vi "CRYTS Step Unflatten Lib.vi"(9 "Version":i32, 10 "Sequence Name":string, 11 "Steps In":T1[](array[typedef]) {"Repeat State Array"."Start" format="%#_5g"; "Y dB ref" format="%.1f"; "Y data" items=["dB", "Lin"]; "Start" format="%#_5g"}) -> (3 "Steps Out":T1[](array[typedef]) {"Repeat State Array"."Start" format="%#_5g"; "Y dB ref" format="%.1f"; "Y data" items=["dB", "Lin"]; "Start" format="%#_5g"})   [LabVIEW 2013]
uses:
  CRYSystem/Typedef Control/CRYStep.ctl
  CRYSystem/Typedef Control/CRYStart Cluster.ctl
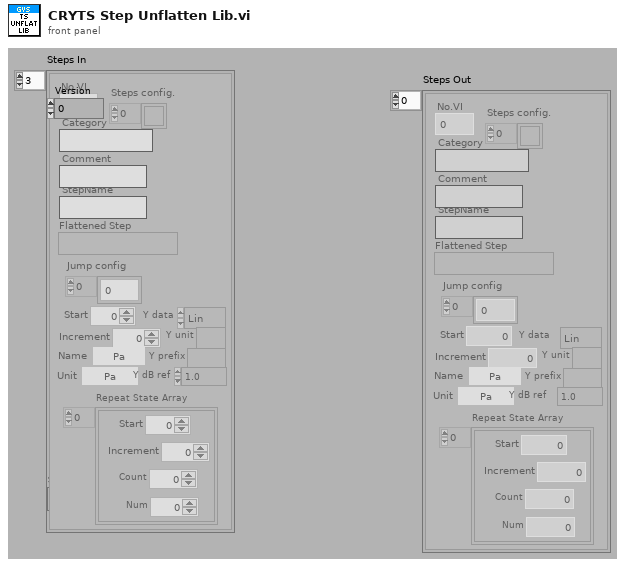
[diagram p1: front panel]
types:
  T1 = typedef "CRYStep.ctl" = cluster{"No.VI":i32, "Category":string, "StepName":string, "Seq setup flattened":string, "Comment":string, "Steps config.":bool[], "Jump config":i32[], "Start":dbl, "Increment":dbl, "Name":string, "Unit":string, "Y data":u16, "Y prefix":string, "Y dB ref":dbl, "Y unit":string, "Repeat State Array":cluster{"Start":dbl, "Increment":dbl, "Count":i32, "Num":i32}[]}
  T2 = typedef "CRYStart Cluster.ctl" = cluster{"SequenceName":string, "Preload Stimulus":bool, "CloseOpenedDisplay":bool, "ClearMeasuredData":bool, "UpdateDisplayDuringRun":bool, "DisplayForConfirmation":bool, "HaltOnFail":bool, "UseSameHardware":bool, "UseSameCalibration":bool}
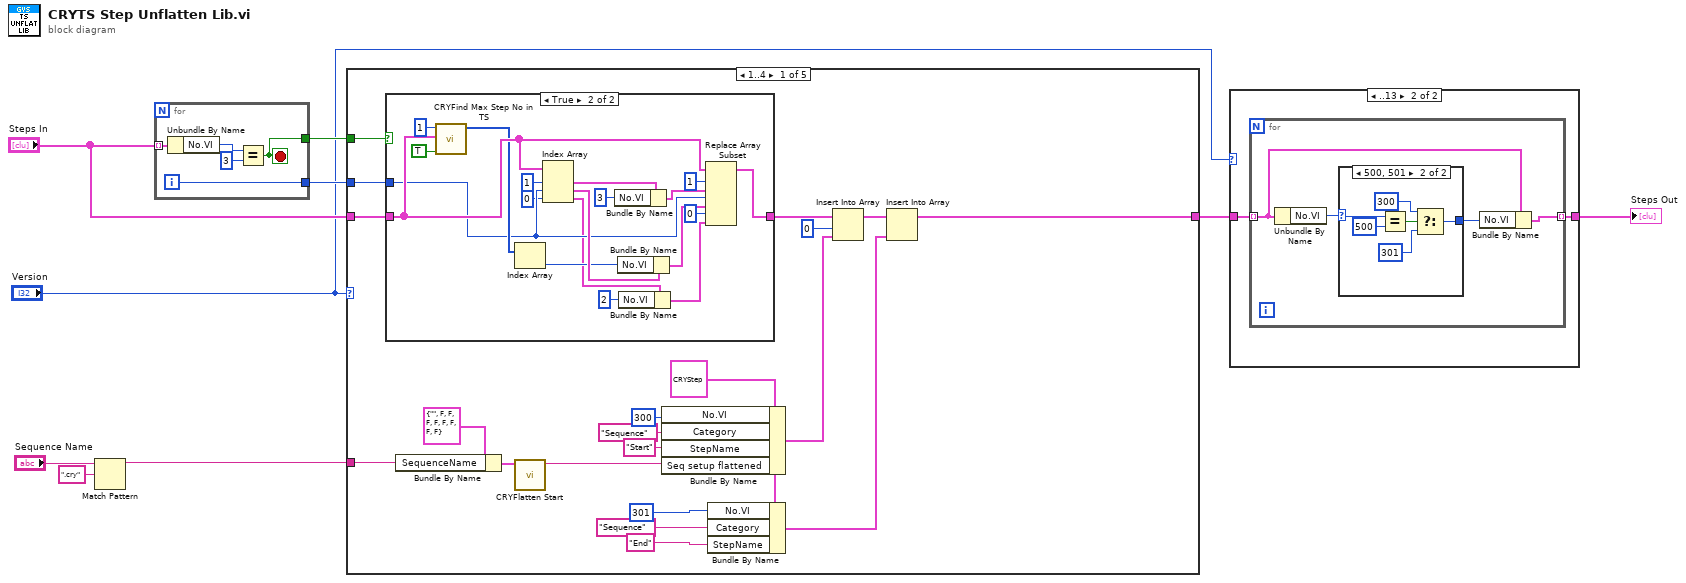
[diagram p0: block diagram]
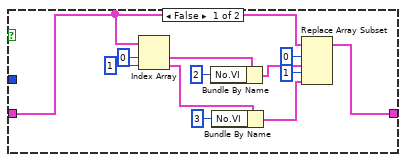
[diagram p4: hidden frame]
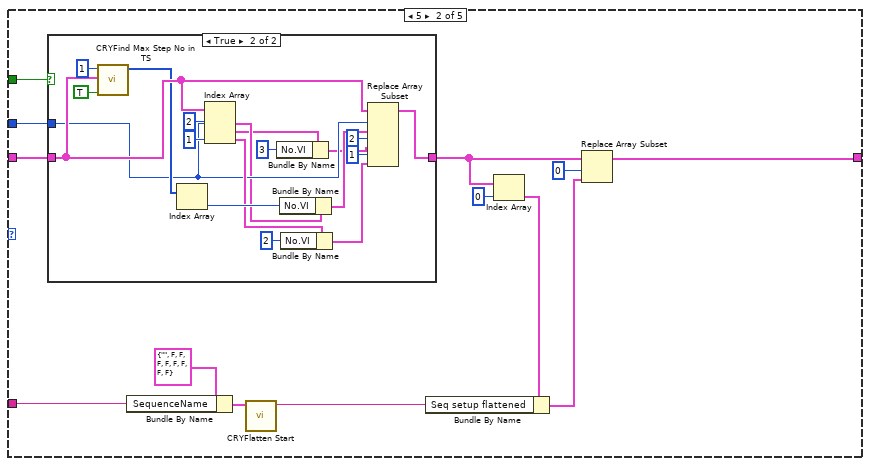
[diagram p5: hidden frame]
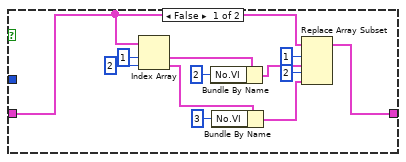
[diagram p6: hidden frame]
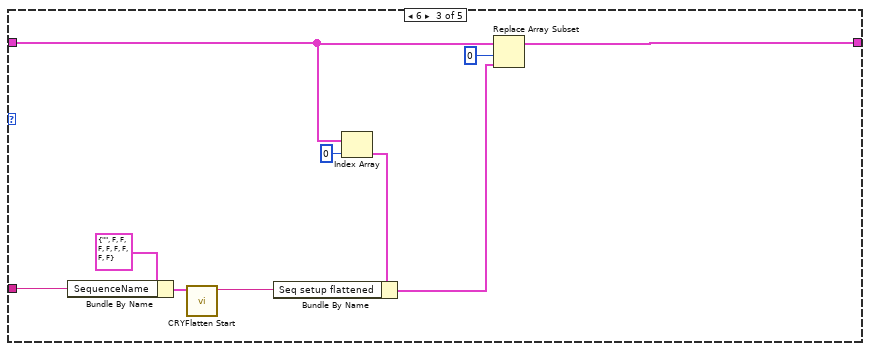
[diagram p7: hidden frame]
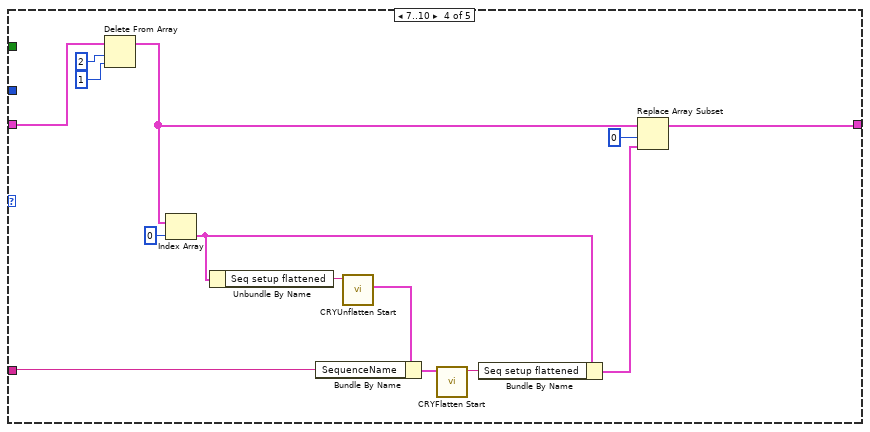
[diagram p8: hidden frame]
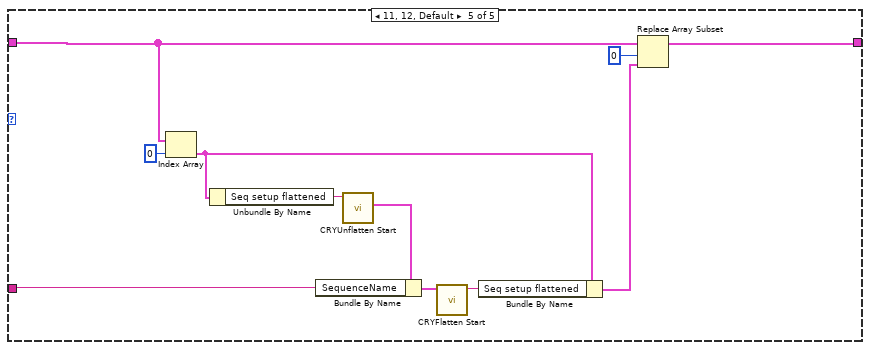
[diagram p9: hidden frame]
diagram:
  n1 = Match Pattern(string="Sequence Name", regular expression=".cry") -> (before substring=w4:string)  [unwired: 1 in, 3 out]
  n2 = for {
    tunnel: "Steps In" -> [w14] mode=indexing
    tunnel: [w11] -> w7
    tunnel: [w10] -> w9
    i -> [w11]
    stop <- w10 stop-if-true
    n3 = Unbundle By Name(w14) -> ("No.VI"=w13:i32)
    n4 = Equal?(x=w13, y=3) -> (x = y?=w10:bool)
  }
  n5 = case shown="1..4" "Version" {
    tunnel: w9 -> [w34 w76 _ _ _]
    tunnel: "Steps In" -> [w33 w78 w115 w123 w134]
    tunnel: w7 -> [w32 w77 _ _ _]
    tunnel: [w19 w70 w114 w130 w141] -> w2
    tunnel: w4 -> [w15 w67 w110 w126 w137]
    frame 1..4 {
      w29 = T1 {"No.VI"=0, "Category"="", "StepName"="", "Seq setup flattened"="", "Comment"="", "Steps config."=[], "Jump config"=[], "Start"=0.0, "Increment"=0.0, "Name"="", "Unit"="", "Y data"=0, "Y prefix"="", "Y dB ref"=0.0, "Y unit"="", "Repeat State Array"=[]} ("Step")
      n6 = case shown="True" w34 {
        tunnel: w33 -> [w42 w58]
        tunnel: [w41 w57] -> w20
        tunnel: w32 -> [_ w53]
        frame False {
          n7 = Index Array(array=w42, index #1=0 ("index"), index #2=1 ("index")) -> (element #1=w37:T1, element #2=w35:T1)
          n8 = Bundle By Name(cluster=w37, "No.VI"=2) -> (w46:T1)
          n9 = Bundle By Name(cluster=w35, "No.VI"=3) -> (w36:T1)
          n10 = Replace Array Subset(array=w42, new element #1=w46, index #1=0 ("index"), new element #2=w36, index #2=1 ("index")) -> (w41:T1[])
        }
        frame True {
          n11 = call "CRYFind Max Step No in TS.vi"("Inputflg"=TRUE, "Steps In"=w58, "Required Count"=1) -> ("Num Array Out"=w55:i32[])  [unwired: 8 in]
          n12 = Index Array(array=w55) -> (element=w54:i32)  [unwired: 1 in]
          n13 = Index Array(array=w58, index #1=1 ("index"), index #2=w53, index #3=0 ("index")) -> (element #1=w60:T1, element #2=w56:T1, element #3=w49:T1)
          n14 = Bundle By Name(cluster=w60, "No.VI"=3) -> (w63:T1)
          n15 = Bundle By Name(cluster=w56, "No.VI"=w54) -> (w52:T1)
          n16 = Bundle By Name(cluster=w49, "No.VI"=2) -> (w48:T1)
          n17 = Replace Array Subset(array=w58, new element #1=w63, index #1=1 ("index"), new element #2=w52, index #2=w53, new element #3=w48, index #3=0 ("index")) -> (w57:T1[])
        }
      }
      n18 = Bundle By Name(cluster=T2 {"SequenceName"="", "Preload Stimulus"=FALSE, "CloseOpenedDisplay"=FALSE, "ClearMeasuredData"=FALSE, "UpdateDisplayDuringRun"=FALSE, "DisplayForConfirmation"=FALSE, "HaltOnFail"=FALSE, "UseSameHardware"=FALSE, "UseSameCalibration"=FALSE} ("Sequence Configure"), "SequenceName"=w15) -> (w18:T2)
      n19 = call "CRYFlatten Start.vi"("Start"=w18) -> ("Start flattened"=w16:string)  [unwired: 10 in]
      n20 = Bundle By Name(cluster=w29, "No.VI"=300, "Category"="Sequence", "StepName"="Start" ("Category"), "Seq setup flattened"=w16) -> (w27:T1)
      n21 = Bundle By Name(cluster=w29, "No.VI"=301, "Category"="Sequence", "StepName"="End" ("Category")) -> (w28:T1)
      n22 = Insert Into Array(array=w20, index=0, new element=w27) -> (w31:T1[])
      n23 = Insert Into Array(array=w31, new element=w28) -> (w19:T1[])  [unwired: 1 in]
    }
    frame 5 {
      n24 = case shown="True" w76 {
        tunnel: w78 -> [w86 w106]
        tunnel: [w85 w105] -> w73
        tunnel: w77 -> [_ w97]
        frame False {
          n25 = Index Array(array=w86, index #1=1 ("index"), index #2=2 ("index")) -> (element #1=w81:T1, element #2=w79:T1)
          n26 = Bundle By Name(cluster=w81, "No.VI"=2) -> (w90:T1)
          n27 = Bundle By Name(cluster=w79, "No.VI"=3) -> (w80:T1)
          n28 = Replace Array Subset(array=w86, new element #1=w90, index #1=1 ("index"), new element #2=w80, index #2=2 ("index")) -> (w85:T1[])
        }
        frame True {
          n29 = call "CRYFind Max Step No in TS.vi"("Inputflg"=TRUE, "Steps In"=w106, "Required Count"=1) -> ("Num Array Out"=w104:i32[])  [unwired: 8 in]
          n30 = Index Array(array=w104) -> (element=w103:i32)  [unwired: 1 in]
          n31 = Index Array(array=w106, index #1=w97, index #2=2 ("index"), index #3=1 ("index")) -> (element #1=w95:T1, element #2=w93:T1, element #3=w100:T1)
          n32 = Bundle By Name(cluster=w93, "No.VI"=3) -> (w91:T1)
          n33 = Bundle By Name(cluster=w95, "No.VI"=w103) -> (w96:T1)
          n34 = Bundle By Name(cluster=w100, "No.VI"=2) -> (w99:T1)
          n35 = Replace Array Subset(array=w106, new element #1=w96, index #1=w97, new element #2=w91, index #2=2 ("index"), new element #3=w99, index #3=1 ("index")) -> (w105:T1[])
        }
      }
      n36 = Bundle By Name(cluster=T2 {"SequenceName"="", "Preload Stimulus"=FALSE, "CloseOpenedDisplay"=FALSE, "ClearMeasuredData"=FALSE, "UpdateDisplayDuringRun"=FALSE, "DisplayForConfirmation"=FALSE, "HaltOnFail"=FALSE, "UseSameHardware"=FALSE, "UseSameCalibration"=FALSE} ("Sequence Configure"), "SequenceName"=w67) -> (w69:T2)
      n37 = call "CRYFlatten Start.vi"("Start"=w69) -> ("Start flattened"=w66:string)  [unwired: 10 in]
      n38 = Index Array(array=w73, index=0) -> (element=w74:T1)
      n39 = Bundle By Name(cluster=w74, "Seq setup flattened"=w66) -> (w71:T1)
      n40 = Replace Array Subset(array=w73, new element=w71, index=0) -> (w70:T1[])
    }
    frame 6 {
      n41 = Bundle By Name(cluster=T2 {"SequenceName"="", "Preload Stimulus"=FALSE, "CloseOpenedDisplay"=FALSE, "ClearMeasuredData"=FALSE, "UpdateDisplayDuringRun"=FALSE, "DisplayForConfirmation"=FALSE, "HaltOnFail"=FALSE, "UseSameHardware"=FALSE, "UseSameCalibration"=FALSE} ("Sequence Configure"), "SequenceName"=w110) -> (w113:T2)
      n42 = call "CRYFlatten Start.vi"("Start"=w113) -> ("Start flattened"=w111:string)  [unwired: 10 in]
      n43 = Index Array(array=w115, index=0) -> (element=w118:T1)
      n44 = Bundle By Name(cluster=w118, "Seq setup flattened"=w111) -> (w116:T1)
      n45 = Replace Array Subset(array=w115, new element=w116, index=0) -> (w114:T1[])
    }
    frame 7..10 {
      n46 = Delete From Array(array=w123, length=2, index=1) -> (array with subset deleted=w120:T1[])  [unwired: 1 out]
      n47 = Index Array(array=w120, index=0) -> (element=w129:T1)
      n48 = Unbundle By Name(w129) -> ("Seq setup flattened"=w128:string)
      n49 = call "CRYUnflatten Start.vi"("Unflatten Sequence"=w128) -> ("Sequence Configure"=w127:T2)  [unwired: 8 in, 2 out]
      n50 = Bundle By Name(cluster=w127, "SequenceName"=w126) -> (w125:T2)
      n51 = call "CRYFlatten Start.vi"("Start"=w125) -> ("Start flattened"=w124:string)  [unwired: 10 in]
      n52 = Bundle By Name(cluster=w129, "Seq setup flattened"=w124) -> (w131:T1)
      n53 = Replace Array Subset(array=w120, new element=w131, index=0) -> (w130:T1[])
    }
    frame 11, 12, Default {
      n54 = Index Array(array=w134, index=0) -> (element=w140:T1)
      n55 = Unbundle By Name(w140) -> ("Seq setup flattened"=w139:string)
      n56 = call "CRYUnflatten Start.vi"("Unflatten Sequence"=w139) -> ("Sequence Configure"=w138:T2)  [unwired: 8 in, 2 out]
      n57 = Bundle By Name(cluster=w138, "SequenceName"=w137) -> (w136:T2)
      n58 = call "CRYFlatten Start.vi"("Start"=w136) -> ("Start flattened"=w135:string)  [unwired: 10 in]
      n59 = Bundle By Name(cluster=w140, "Seq setup flattened"=w135) -> (w142:T1)
      n60 = Replace Array Subset(array=w134, new element=w142, index=0) -> (w141:T1[])
    }
  }
  n61 = case shown="..13" "Version" {
    tunnel: w2 -> [w145 w147]
    tunnel: [w145 w146] -> w1
    frame Default {
    }
    frame ..13 {
      n62 = for {
        tunnel: w147 -> [w150] mode=indexing
        tunnel: [w148] -> w146 mode=indexing
        n63 = Unbundle By Name(w150) -> ("No.VI"=w151:i32)
        n64 = case shown="500, 501" w151 {
          selector: w151 -> [w152 w158]
          tunnel: [w152 w155] -> w149
          frame Default {
          }
          frame 500, 501 {
            n65 = Equal?(x=w158, y=500) -> (x = y?=w156:bool)
            n66 = Select(t=300 ("y"), s=w156, f=301) -> (s? t:f=w155:i32)
          }
        }
        n67 = Bundle By Name(cluster=w150, "No.VI"=w149) -> (w148:T1)
      }
    }
  }
  "Steps Out" <- w1
